vi "String - Convert SQL Date (YYYY-mm-dd) to UserDefined Date.vi"(7 "Date Format (UserDefined)":string, 8 "Error In":errorcluster, 11 "YYYY-mm-dd":string) -> (0 "error out":errorcluster, 3 "Date String (UserDefined)":string)   [LabVIEW 2013]
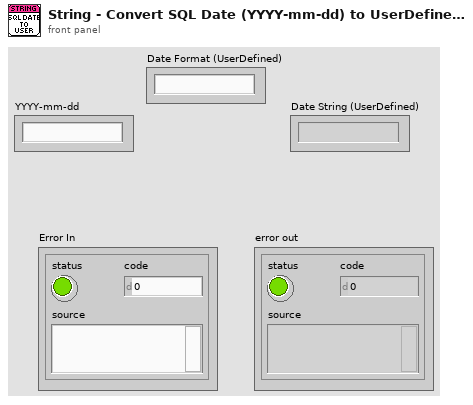
[diagram p1: front panel]
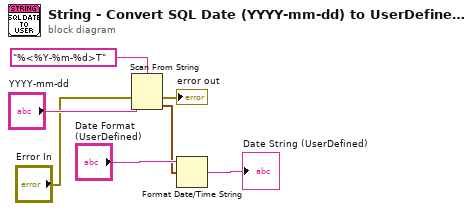
[diagram p0: block diagram]
diagram:
  n1 = Scan From String(format string="%<%Y-%m-%d>T", input string="YYYY-mm-dd", error in="Error In") -> (error out=→"error out":errorcluster, output 1=w6:timestamp)  [unwired: 2 in, 2 out]
  n2 = Format Date/Time String(time format string (%c)="Date Format (UserDefined)", seconds (now)=w6) -> (date/time string=→"Date String (UserDefined)":string)  [unwired: 1 in]
